vi "obtainSALLVFunctionReferences.vi"(8 "error in (no error)":errorcluster, 11 "summaryState in":refnum<class "summaryState.lvclass">) -> (0 "error out":errorcluster, 3 "summaryState out":refnum<class "summaryState.lvclass">)   [LabVIEW 2016, in "SALLV_AtDome_Messaging.lvlib" / "summaryState.lvclass"]
uses:
  summaryState.lvclass
  home/andres/ts_AtDome/SALTopic/SALTopic/SALTopic.lvclass
  summaryState.lvclass/summaryState.ctl
  SALTopic/SALEvent/SALEvent.lvclass
  SALTopic/SALTopic/SALTopic.lvclass
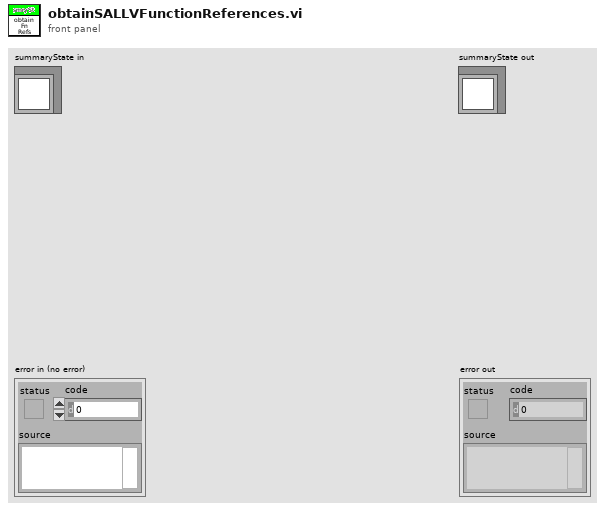
[diagram p1: front panel]
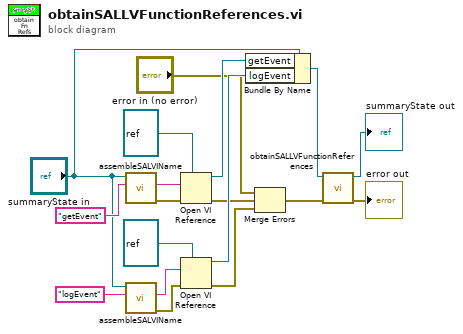
[diagram p0: block diagram]
diagram:
  n1 = call "assembleSALVIName.vi"("topicKey"="getEvent" ("commandKey"), "SALTopic in"="summaryState in") -> ("error out"=w14:errorcluster, "viPath"=w15:string)  [unwired: 7 in, 1 out]
  n2 = call "assembleSALVIName.vi"("topicKey"="logEvent" ("commandKey"), "SALTopic in"="summaryState in") -> ("error out"=w11:errorcluster, "viPath"=w10:string)  [unwired: 7 in, 1 out]
  n3 = Open VI Reference(type specifier VI Refnum (for type only)=refnum<vi> refnum ("reference"), vi path=w15, error in (no error)=w14) -> (vi reference=w7:refnum<vi>, error out=w3:errorcluster)  [unwired: 3 in]
  n4 = Open VI Reference(type specifier VI Refnum (for type only)=refnum<vi> refnum ("reference"), vi path=w10, error in (no error)=w11) -> (vi reference=w6:refnum<vi>, error out=w2:errorcluster)  [unwired: 3 in]
  n5 = Bundle By Name(cluster="summaryState in", "getEvent"=w7, "logEvent"=w6) -> (w5:refnum<class "summaryState.lvclass">)
  n6 = Merge Errors("error in (no error)", w3, w2) -> (w1:errorcluster)
  n7 = call-parent "obtainSALLVFunctionReferences.vi"("error in (no error)"=w1, "SALEvent in"=w5) -> ("error out"=→"error out":errorcluster, "SALEvent out"=→"summaryState out":refnum<class "summaryState.lvclass">)  [unwired: 8 in]
